vi "close socket.vi"(8 "error in (no error)":errorcluster, 11 "Communication Channel in":refnum<class "Communication Channel.lvclass">) -> (0 "error out":errorcluster, 3 "Communication Channel out":refnum<class "Communication Channel.lvclass">)   [LabVIEW 2018, in "Communication Channel.lvclass"]
uses:
  Communication Channel.lvclass
  Socket/Socket.lvclass
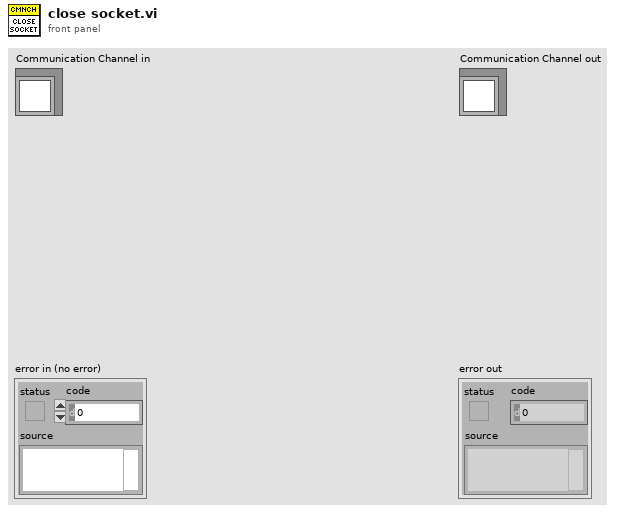
[diagram p1: front panel]
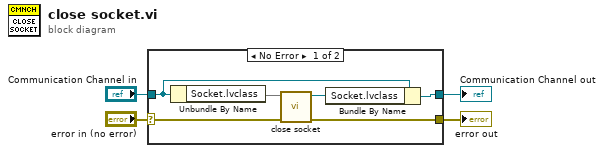
[diagram p0: block diagram]
diagram:
  n1 = case shown="No Error" "error in (no error)" {
    selector: "error in (no error)" -> [w9 w12]
    tunnel: [w8 w12] -> w3
    tunnel: [w5 w11] -> w1
    tunnel: "Communication Channel in" -> [w7 w11]
    frame No Error {
      n2 = Unbundle By Name(w7) -> ("Socket.lvclass"=w10)
      n3 = call "close socket.vi"("error in (no error)"=w9, "Socket in"=w10) -> ("error out"=w8:errorcluster, "Socket out"=w6:refnum<class "Socket.lvclass">)  [unwired: 8 in]
      n4 = Bundle By Name(cluster=w7, "Socket.lvclass"=w6) -> (w5:refnum<class "Communication Channel.lvclass">)
    }
    frame Error {
    }
  }
  "error out" <- w3
  "Communication Channel out" <- w1
